vi "read_settings.vi"(8 "error in (no error)":errorcluster) -> (0 "error out":errorcluster)   [LabVIEW 2017]
doc: "reads the settings from the settings.ini"
uses:
  <vilib>/Utility/config.llb/Read Key (String).vi
  global_variables.vi
  <vilib>/Utility/config.llb/Read Key (Path).vi
  <vilib>/Utility/config.llb/NI_LVConfig.lvlib
panel:
  out "appended path":path
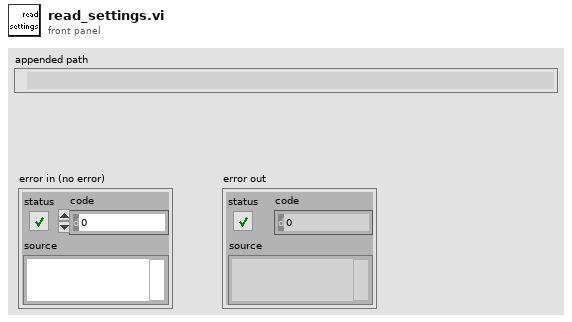
[diagram p1: front panel]
types:
  T1 = typedef "NI_LVConfig.lvlib/Config Data RefNum.ctl" = refnum<k1>
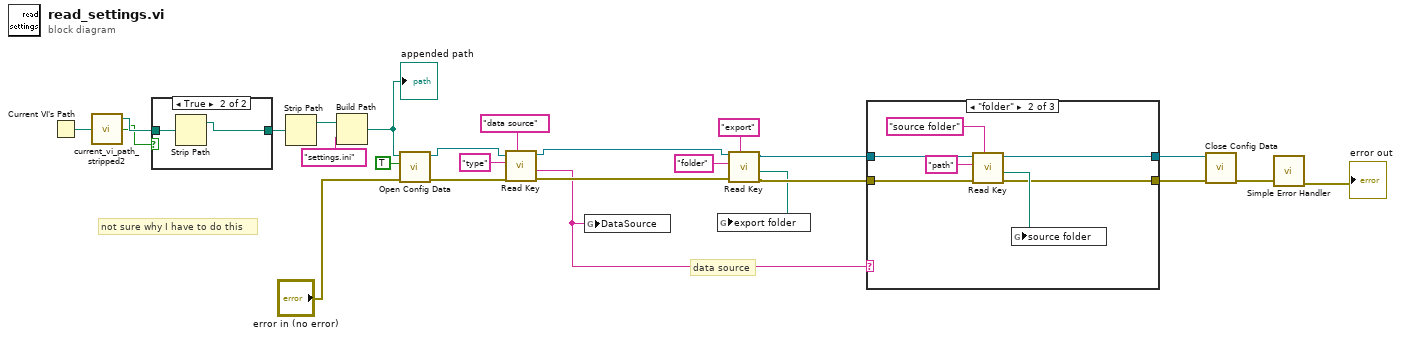
[diagram p0: block diagram]
diagram:
  # "data source"
  # "not sure why I have to do this"
  n1 = Current VI's Path() -> (path=w15:path)
  n2 = call "current_vi_path_stripped2.vi"("current VI Path"=w15) -> ("exe?"=w12:bool, "current VI Path stripped out"=w13:path)  [unwired: 3 in]
  n3 = case shown="True" w12 {
    tunnel: [w26 w27] -> w14
    tunnel: w13 -> [w26 w28]
    frame False {
    }
    frame True {
      n4 = Strip Path(path=w28) -> (stripped path=w27:path)  [unwired: 1 out]
    }
  }
  n5 = Strip Path(path=w14) -> (stripped path=w16:path)  [unwired: 1 out]
  n6 = Build Path(base path=w16, name or relative path="settings.ini") -> (appended path=w23:path)
  "appended path" <- w23
  n7 = call <vilib>:"Open Config Data.vi"("error in (no error)"="error in (no error)", "create file if necessary (T)"=TRUE, "configuration file path"=w23) -> ("error out"=w8:errorcluster, "refnum"=w9:T1)  [unwired: 6 in, 1 out]
  n8 = call-poly <vilib>:"Read Key.vi"("section"="data source", "error in (no error)"=w8, "key"="type", "refnum"=w9) -> ("error out"=w6:errorcluster, "value"=w5:string, "refnum out"=w7:T1)  [unwired: 4 in, 1 out]
  n9 = global write "global_variables.vi" "DataSource"(w5) -> ()
  n10 = call-poly <vilib>:"Read Key.vi"("section"="export", "error in (no error)"=w6, "key"="folder", "refnum"=w7) -> ("error out"=w20:errorcluster, "value"=w19:path, "refnum out"=w21:T1)  [unwired: 4 in, 1 out]
  n11 = global write "global_variables.vi" "export folder"(w19) -> ()
  n12 = case shown="\"folder\"" w5 {
    tunnel: w21 -> [w30 w36 w39]
    tunnel: w20 -> [w29 w35 w38]
    tunnel: [w29 w31 w38] -> w4
    tunnel: [w30 w33 w39] -> w3
    frame "False", Default {
    }
    frame "folder" {
      n13 = call-poly <vilib>:"Read Key.vi"("section"="source folder", "error in (no error)"=w35, "key"="path", "refnum"=w36) -> ("error out"=w31:errorcluster, "value"=w34:path, "refnum out"=w33:T1)  [unwired: 4 in, 1 out]
      n14 = global write "global_variables.vi" "source folder"(w34) -> ()
    }
    frame "database" {
    }
  }
  n15 = call <vilib>:"Close Config Data.vi"("error in (no error)"=w4, "refnum"=w3) -> ("error out"=w2:errorcluster)  [unwired: 8 in, 1 out]
  n16 = call <vilib>:"Simple Error Handler.vi"("error in (no error)"=w2) -> ("error out"=→"error out":errorcluster)  [unwired: 4 in, 4 out]
